vi "Bool_toStr.vi"(11 "znaleziono?":bool) -> (3 "String":string)   [LabVIEW 2014]
doc: "Konwertuje zmienną boolinową \ndo stringa \"T\" lub \"F\""
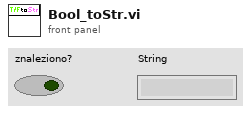
[diagram p1: front panel]
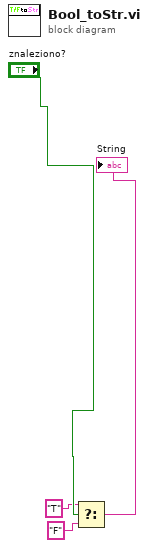
[diagram p0: block diagram]
diagram:
  n1 = Select(t="T", s="znaleziono?", f="F") -> (s? t:f=→"String":string)
